vi "Read PV Connections.vi"(8 "error in (no error)":errorcluster, 11 "CS++PVMonitor in":refnum<class "CS++PVMonitor.lvclass">) -> (0 "error out":errorcluster, 2 "PV Connections":T1(array[cluster]), 3 "CS++PVMonitor out":refnum<class "CS++PVMonitor.lvclass">)   [LabVIEW 2015, in "CS++PVMonitor.lvlib" / "CS++PVMonitor.lvclass"]
doc: "Read PV connections."
uses:
  CS++PVMonitor.lvclass
  <vilib>/ActorFramework/Message Enqueuer/Message Enqueuer.lvclass
  CS++PVMonitor Messages/CS++PVUpdate Msg/CS++PVUpdate Msg.lvclass
  CS++PVMonitor.lvclass/CS++PVMonitor.ctl
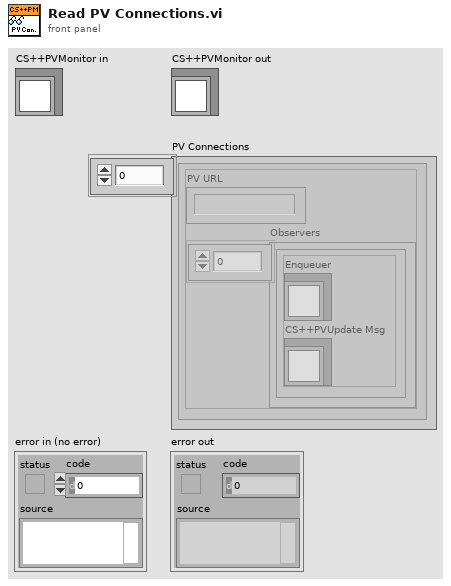
[diagram p1: front panel]
types:
  T1 = cluster{"PV URL":string, "Observers":cluster{"Enqueuer":refnum<class "Message Enqueuer.lvclass">, "CS++PVUpdate Msg":refnum<class "CS++PVUpdate Msg.lvclass">}[]}[]
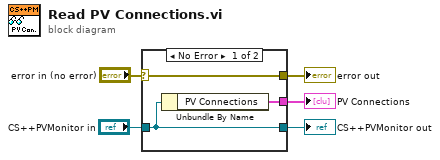
[diagram p0: block diagram]
diagram:
  n1 = case shown="No Error" "error in (no error)" {
    selector: "error in (no error)" -> [w8 w9]
    tunnel: [w8 w9] -> w4
    tunnel: [w7 w10] -> w2
    tunnel: "CS++PVMonitor in" -> [w7 w10]
    tunnel: [w6 _] -> w1
    frame No Error {
      n2 = Unbundle By Name(w7) -> ("PV Connections"=w6:T1)
    }
    frame Error {
    }
  }
  "error out" <- w4
  "CS++PVMonitor out" <- w2
  "PV Connections" <- w1
